vi "Detect_FTDI-USBSerial.vi"(8 "error in (no error)":errorcluster) -> (0 "error out":errorcluster, 3 "selected comport":string, 5 "# of FTDI Devices":i32, 7 "Success(t)":bool caption="OK")   [LabVIEW 2018]
panel:
  out "Numeric":i32
  out "spreadsheet string":string
  out "Array 2":string[](array[string])
  out "comport_index":dbl
  out "No Devices?(t)":bool
  out "more than1dev?(t)":bool
  out "Comports":string[](array[string])
  out "trimmed string":string[](array[string])
  out "Array":string[][](array[string])
  out "comport indices":i32[](array[numeric])
  out "Device Match Indices":i32[](array[numeric])
  out "Match Values":string[](array[string])
  in  "expected output size  (4096)":u32
  out "standard output":string
  in  "run minimized? (F)":bool
  in  "wait until completion? (T)":bool=TRUE
  in  "working directory":path=path ""
  in  "standard input":string
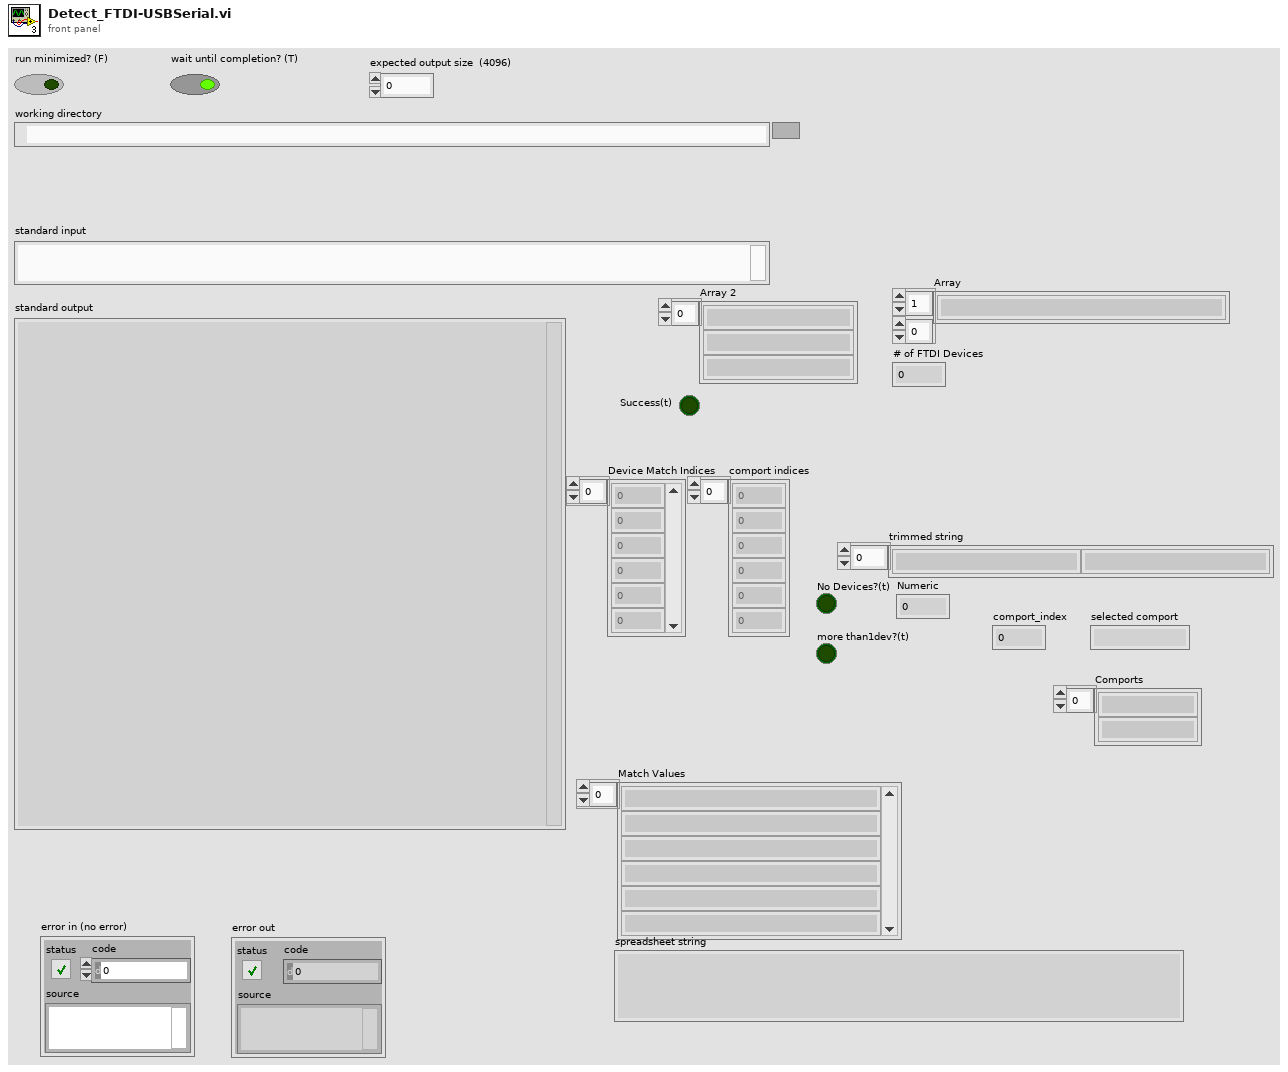
[diagram p1: front panel]
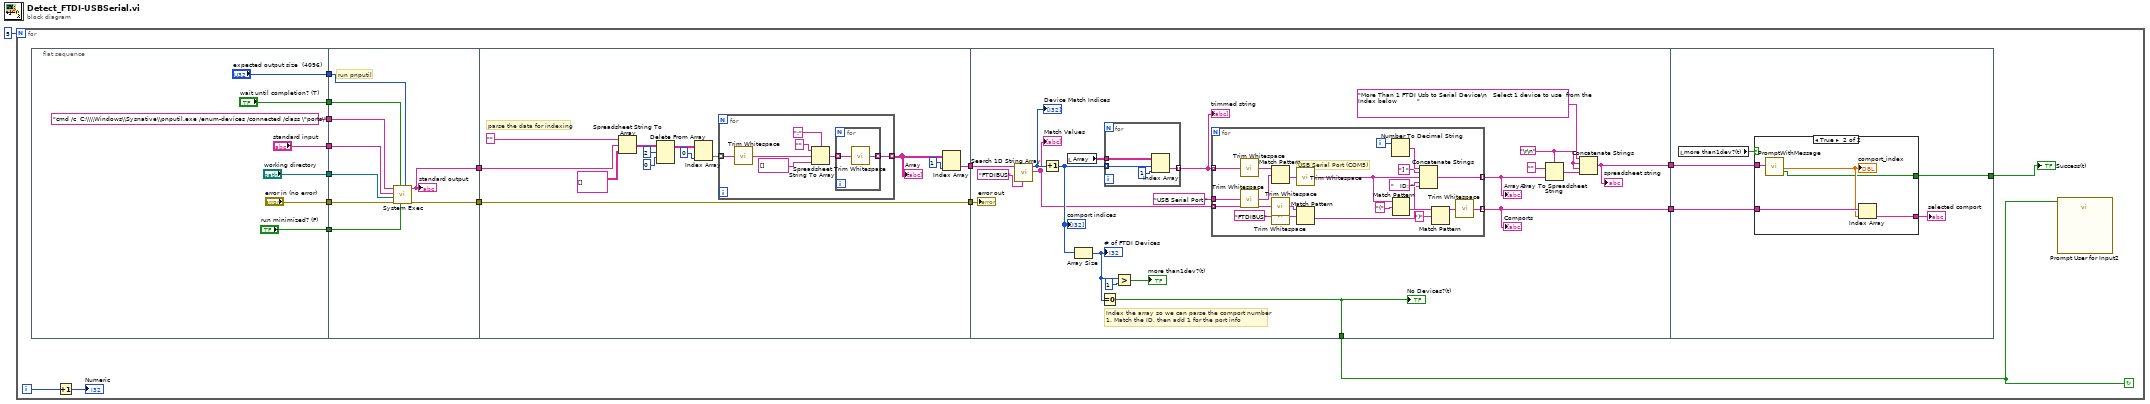
[diagram p0: block diagram]
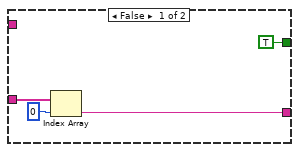
[diagram p2: hidden frame]
diagram:
  n1 = for {
    N: 5 -> [_]
    i -> [w5]
    stop <- w3 continue-if-true
    n2 = flat-sequence {
      tunnel: ["working directory"] -> w18
      tunnel: ["cmd /c  C:\\\\Windows\\Sysnative\\pnputil.exe /enum-devices /connected /class \"ports\"" ("command line")] -> w17
      tunnel: ["standard input"] -> w16
      tunnel: ["wait until completion? (T)"] -> w15
      tunnel: ["run minimized? (F)"] -> w14
      tunnel: ["expected output size  (4096)"] -> w13
      tunnel: ["error in (no error)"] -> w12
      tunnel: w18 -> [w34]
      tunnel: w17 -> [w33]
      tunnel: w16 -> [w32]
      tunnel: w15 -> [w31]
      tunnel: w14 -> [w30]
      tunnel: w13 -> [w29]
      tunnel: w12 -> [w28]
      tunnel: [w27] -> w11
      tunnel: [w26] -> w10
      tunnel: w11 -> [w35]
      tunnel: w10 -> [w38]
      tunnel: [w35] -> w9
      tunnel: [w36] -> w8
      tunnel: w9 -> [w73]
      tunnel: w8 -> [w75]
      tunnel: [w65] -> w7
      tunnel: [w61] -> w6
      tunnel: [w57] -> w3
      tunnel: w7 -> [w106]
      tunnel: w6 -> [w103]
      tunnel: [w102] -> w2
      frame #0 {
      }
      frame #1 {
        # "run pnputil"
        n3 = call <vilib>:"System Exec.vi"("expected output size  (4096)"=w29, "run minimized? (F)"=w30, "wait until completion? (T)"=w31, "error in (no error)"=w28, "working directory"=w34, "standard input"=w32, "command line"=w33) -> ("error out"=w27:errorcluster, "standard output"=w26:string)  [unwired: 1 in, 2 out]
        "standard output" <- w26
      }
      frame #2 {
        # "parse the data for indexing"
        n4 = Spreadsheet String To Array(format string="", spreadsheet string=w38, array type (2D Dbl)=string[][] []) -> (array=w46:string[][])  [unwired: 1 in]
        n5 = Delete From Array(array=w46, length=2, index (row)=0) -> (array with subset deleted=w45:string[][])  [unwired: 1 in, 1 out]
        n6 = Index Array(array=w45, index (col)=0 ("disabled index (col)")) -> (element=w44:string[])  [unwired: 1 in]
        n7 = for {
          tunnel: w44 -> [w54] mode=indexing
          tunnel: [w48] -> w47 mode=indexing
          n8 = call <vilib>:"Trim Whitespace.vi"("string"=w54) -> ("trimmed string"=w50:string)  [unwired: 1 in]
          n9 = Spreadsheet String To Array(delimiter (Tab)=":", format string="", spreadsheet string=w50, array type (2D Dbl)=string[] []) -> (array=w49:string[])
          n10 = for {
            tunnel: w49 -> [w56] mode=indexing
            tunnel: [w55] -> w48 mode=indexing
            n11 = call <vilib>:"Trim Whitespace.vi"("string"=w56) -> ("trimmed string"=w55:string)  [unwired: 1 in]
          }
        }
        "Array" <- w47
        n12 = Index Array(array=w47, index (col)=1 ("disabled index (col)")) -> (element=w36:string[])  [unwired: 1 in]
      }
      frame #3 {
        w58 = "\r\n" ("delimiter (Tab)")
        # "Index the array so we can parse the comport number\n1. Match the ID, then add 1 for the port info"
        n13 = call "Search 1D String Array.vi"("Search Term"="FTDIBUS", "Input Array"=w75) -> ("Match Values"=w60:string[], "Match Indices"=w74:i32[])  [unwired: 7 in, 1 out]
        "Match Values" <- w60
        "Device Match Indices" <- w74
        n14 = Increment(x=w74) -> (x+1=w71:i32[])
        "comport indices" <- w71
        n15 = local read "Array"() -> (w72:string[][])
        n16 = Array Size(array=w71) -> (size(s)=w66:i32)
        "# of FTDI Devices" <- w66
        n17 = Equal To 0?(x=w66) -> (x = 0?=w57:bool)
        "No Devices?(t)" <- w57
        n18 = for {
          tunnel: w72 -> [w101]
          tunnel: w71 -> [w100] mode=indexing
          tunnel: [w99] -> w70 mode=indexing
          n19 = Index Array(array=w101, index (row)=w100, index (col)=1 ("disabled index (col)")) -> (element=w99:string)
        }
        "trimmed string" <- w70
        n20 = Greater?(x=w66, y=1) -> (0:→"more than1dev?(t)":bool)
        n21 = for {
          tunnel: w70 -> [w97] mode=indexing
          tunnel: "USB Serial Port " ("regular expression") -> [w96]
          tunnel: [w89] -> w65 mode=indexing
          tunnel: [w86] -> w64 mode=indexing
          tunnel: w60 -> [w81] mode=indexing
          i -> [w87]
          # "USB Serial Port (COM5)"
          n22 = call <vilib>:"Trim Whitespace.vi"("string"=w97) -> ("trimmed string"=w93:string)  [unwired: 1 in]
          n23 = call <vilib>:"Trim Whitespace.vi"("string"=w96) -> ("trimmed string"=w92:string)  [unwired: 1 in]
          n24 = Match Pattern(string=w93, regular expression=w92) -> (after substring=w95:string)  [unwired: 1 in, 3 out]
          n25 = call <vilib>:"Trim Whitespace.vi"("string"=w81) -> ("trimmed string"=w78:string)  [unwired: 1 in]
          n26 = call <vilib>:"Trim Whitespace.vi"("string"="FTDIBUS" ("regular expression")) -> ("trimmed string"=w77:string)  [unwired: 1 in]
          n27 = call <vilib>:"Trim Whitespace.vi"("string"=w95) -> ("trimmed string"=w83:string)  [unwired: 1 in]
          n28 = Match Pattern(string=w78, regular expression=w77) -> (after substring=w79:string)  [unwired: 1 in, 3 out]
          n29 = Number To Decimal String(number=w87) -> (decimal integer string=w85:string)  [unwired: 1 in]
          n30 = Match Pattern(string=w83, regular expression="(") -> (after substring=w94:string)  [unwired: 1 in, 3 out]
          n31 = Concatenate Strings(w85, "] " ("string"), w83, "   ID: " ("string"), w79) -> (w86:string)
          n32 = Match Pattern(string=w94, regular expression=")") -> (before substring=w88:string)  [unwired: 1 in, 3 out]
          n33 = call <vilib>:"Trim Whitespace.vi"("string"=w88) -> ("trimmed string"=w89:string)  [unwired: 1 in]
        }
        "Comports" <- w65
        "Array 2" <- w64
        n34 = Array To Spreadsheet String(delimiter (Tab)=w58, array=w64, 3:"" ("format string")) -> (spreadsheet string=w59:string)
        n35 = Concatenate Strings("More Than 1 FTDI Usb to Serial Device\n   Select 1 device to use  from the Index below          " ("string"), w58, w58, w59) -> (w61:string)
        "spreadsheet string" <- w61
        "error out" <- w73
      }
      frame #4 {
        n36 = local read "more than1dev?(t)"() -> (w104:bool)
        n37 = case shown="True" w104 {
          tunnel: w106 -> [w110 w115]
          tunnel: [w109 w114] -> w105
          tunnel: w103 -> [_ w113]
          tunnel: [TRUE ("OK") w111] -> w102
          frame False {
            n38 = Index Array(array=w110, index=0) -> (element=w109:string)
          }
          frame True {
            n39 = call "PromptWithMessage.vi"("String"=w113) -> ("Index"=w112:dbl, "OK"=w111:bool)  [unwired: 16 in, 1 out]
            "comport_index" <- w112
            n40 = Index Array(array=w115, index=w112) -> (element=w114:string)
          }
        }
        "selected comport" <- w105
      }
    }
    n41 = Increment(x=w5) -> (x+1=→"Numeric":i32)
    n42 = call "Prompt User for Input2"("Enable"=w3) -> ()  [unwired: 17 in, 2 out]
    "Success(t)" <- w2
  }
